vi "Main - Copy.vi"() -> ()   [LabVIEW 2017]
uses:
  <vilib>/addons/database/Connection.llb/Conn ObjectReference.ctl
  <vilib>/addons/database/Connection.llb/DB Tools Open Connec (Path).vi
  Globle/Current date.vi
  <vilib>/addons/database/Connection.llb/Conn Execute.vi
  <vilib>/addons/database/Recordset.llb/Rec Fetch Recordset Data (R).vi
  <vilib>/addons/database/Recordset.llb/Rec Destroy - Connection.vi
  <vilib>/addons/database/NI_Database_API.lvlib
  Globle/Stop.vi
panel:
  out "1D Array":string[](array[string])=["01:00 - 01:59", "02:00 - 02:59", "03:00 - 03:59", "04:00 - 04:59", "05:00 - 05:59", "06:00 - 06:59", "07:00 - 07:59", "08:00 - 08:59", "09:00 - 09:59", "10:00 - 10:59", "11:00 - 11:59", "12:00 - 12:59", "13:00 - 13:59", "14:00 - 14:59", "15:00 - 15:59", "16:00 - 16:59", "17:00 - 17:59", "18:00 - 18:59", "19:00 - 19:59", "20:00 - 20:59", "21:00 - 21:59", "22:00 - 22:59", "22:00 - 22:59", "00:00 - 01:59"]
  out "String Indicator 9":string="BREAKDOWN COUNT"
  out "String Indicator":string="PRODUCTION COUNT"
  out "String Indicator 8":string="REJECTION COUNT"
  out "Dlt Cnt":i32
  out "Table 2":string[][][](array[string])
  out "connection reference":T1
  out "String Indicator 7":string="RUNNING..."
  out "BDWn1":dbl
  out "Rej1":dbl
  out "Prod1":dbl
  out "Total Bdwn Time":timestamp format="%<%H:%M:%S>T"
  out "Hourly1":dbl[](array[numeric])
  out "BSWN3":dbl
  out "Rej3":dbl
  out "Prod 3":dbl
  out "Total Bdwn Time3":timestamp format="%<%H:%M:%S>T"
  out "String Indicator 3":string="RUNNING..."
  out "Hourly3":dbl[](array[numeric])
  out "BDWN2":dbl
  out "Rej2":dbl
  out "Prod 2":dbl
  out "Total Bdwn Time2":timestamp format="%<%H:%M:%S>T"
  out "String Indicator 2":string="RUNNING..."
  out "Hourly2":dbl[](array[numeric])
  out "BDWN6":dbl
  out "Rej6":dbl
  out "Prod6":dbl
  out "Total Bdwn Time4":timestamp format="%<%H:%M:%S>T"
  out "String Indicator 4":string="RUNNING..."
  out "Hourly6":dbl[](array[numeric])
  out "BDWN5":dbl
  out "Rej5":dbl
  out "Prod5":dbl
  out "Total Bdwn Time5":timestamp format="%<%H:%M:%S>T"
  out "String Indicator 5":string="RUNNING..."
  out "Hourly5":dbl[](array[numeric])
  out "BDWN4":dbl
  out "Rej4":dbl
  out "Prod4":dbl
  out "Total Bdwn Time6":timestamp format="%<%H:%M:%S>T"
  out "String Indicator 6":string="RUNNING..."
  out "Hourly4":dbl[](array[numeric])
  out "Numeric Indicator 4":string=" BREAKDOWN TIME "
  out "Numeric Indicator 3":string="STATUS"
  in  "Cancel Button - Archive":bool
  # "Main Screen"
  # "Station_1"
  # "Station_2"
  # "Station_3"
  # "Station_4"
  # "Station_5"
  # "Station_6"
  # "Designed & Developed By: Infinity Automation Systems Pvt. Ltd."
  # "00.00.53\n00.00.25\n00.00.21\n00.00.15\n11\n7\n2\n8\n1.6\n49\n35\n32\n27"
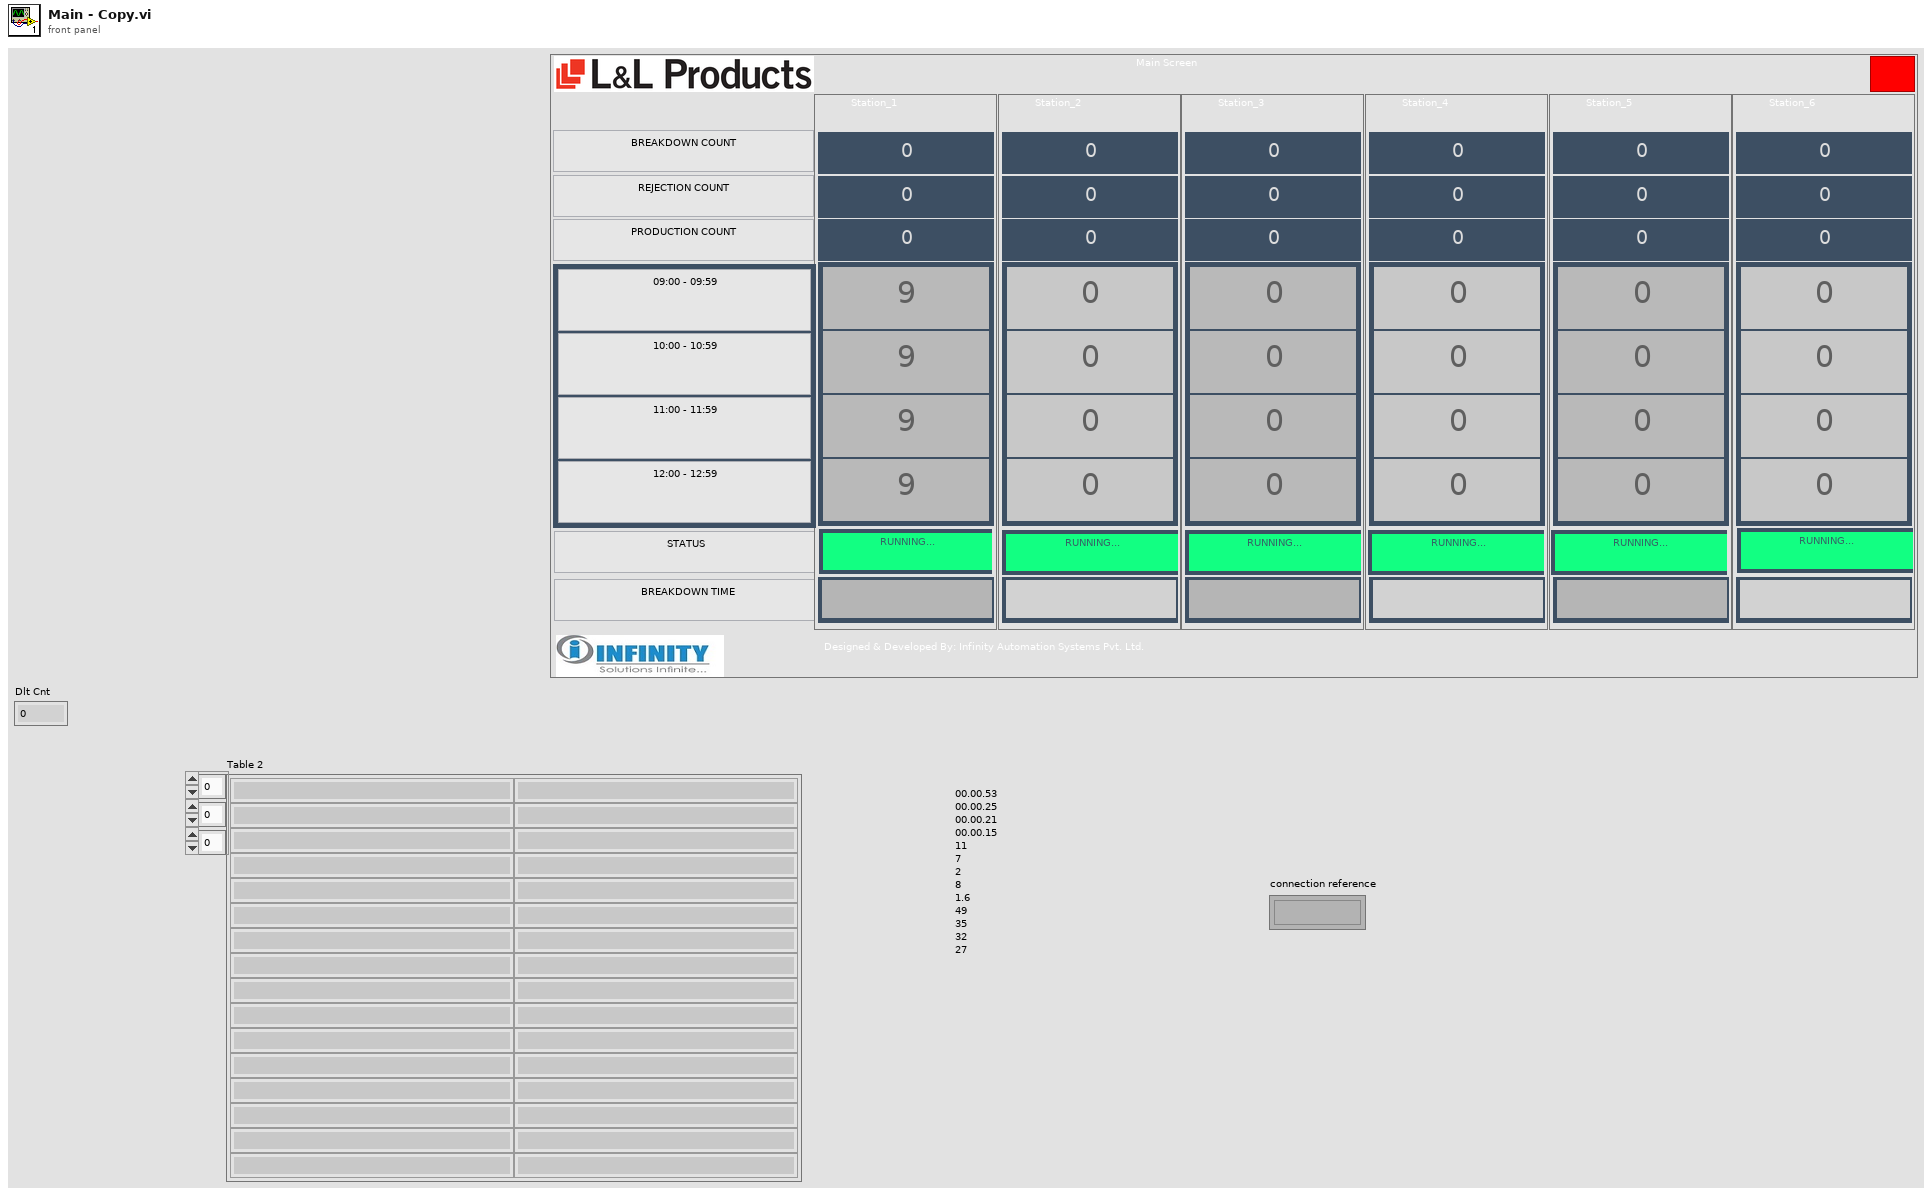
[diagram p1: front panel]
types:
  T1 = typedef "NI_Database_API.lvlib/Conn ObjectReference.ctl" = refnum<k1>
  T2 = typedef "NI_Database_API.lvlib/Rec ObjectReference.ctl" = refnum<k1>
  T3 = enum32{"invalid app kind", "Development System", "Run Time System", "Student Edition", "Embedded LabVIEW", "Evaluation", "Custom"}
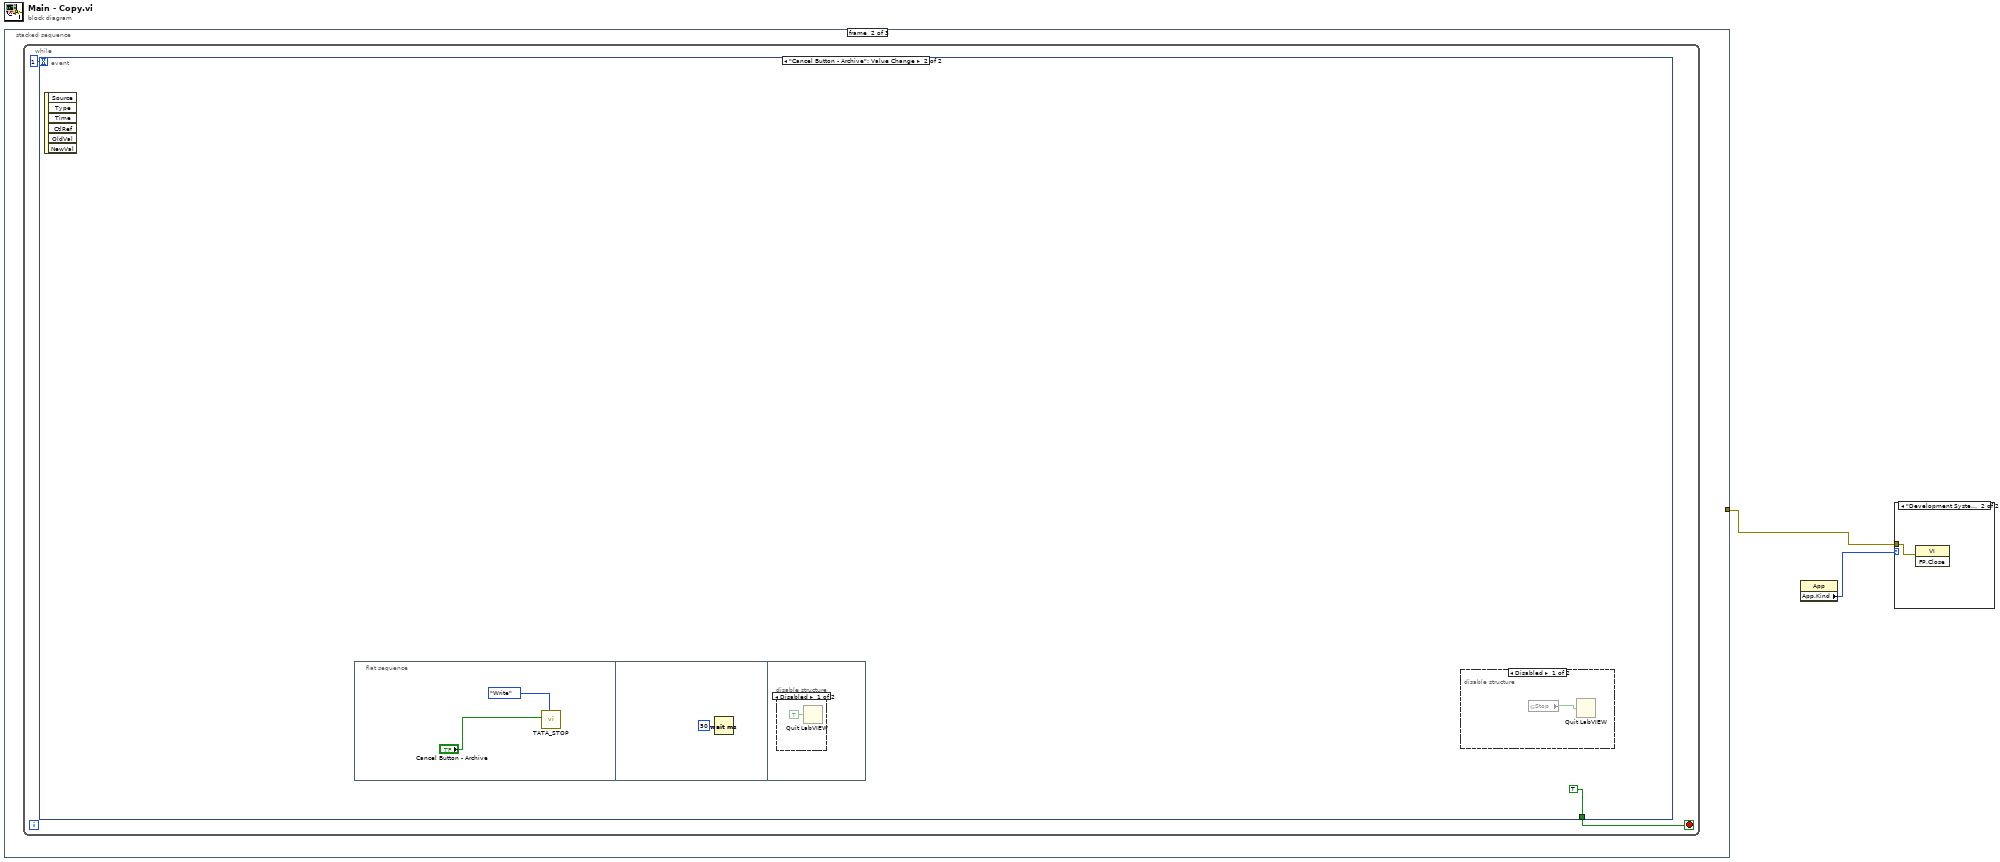
[diagram p0: block diagram]
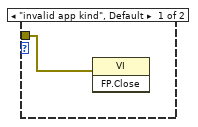
[diagram p2: hidden frame]
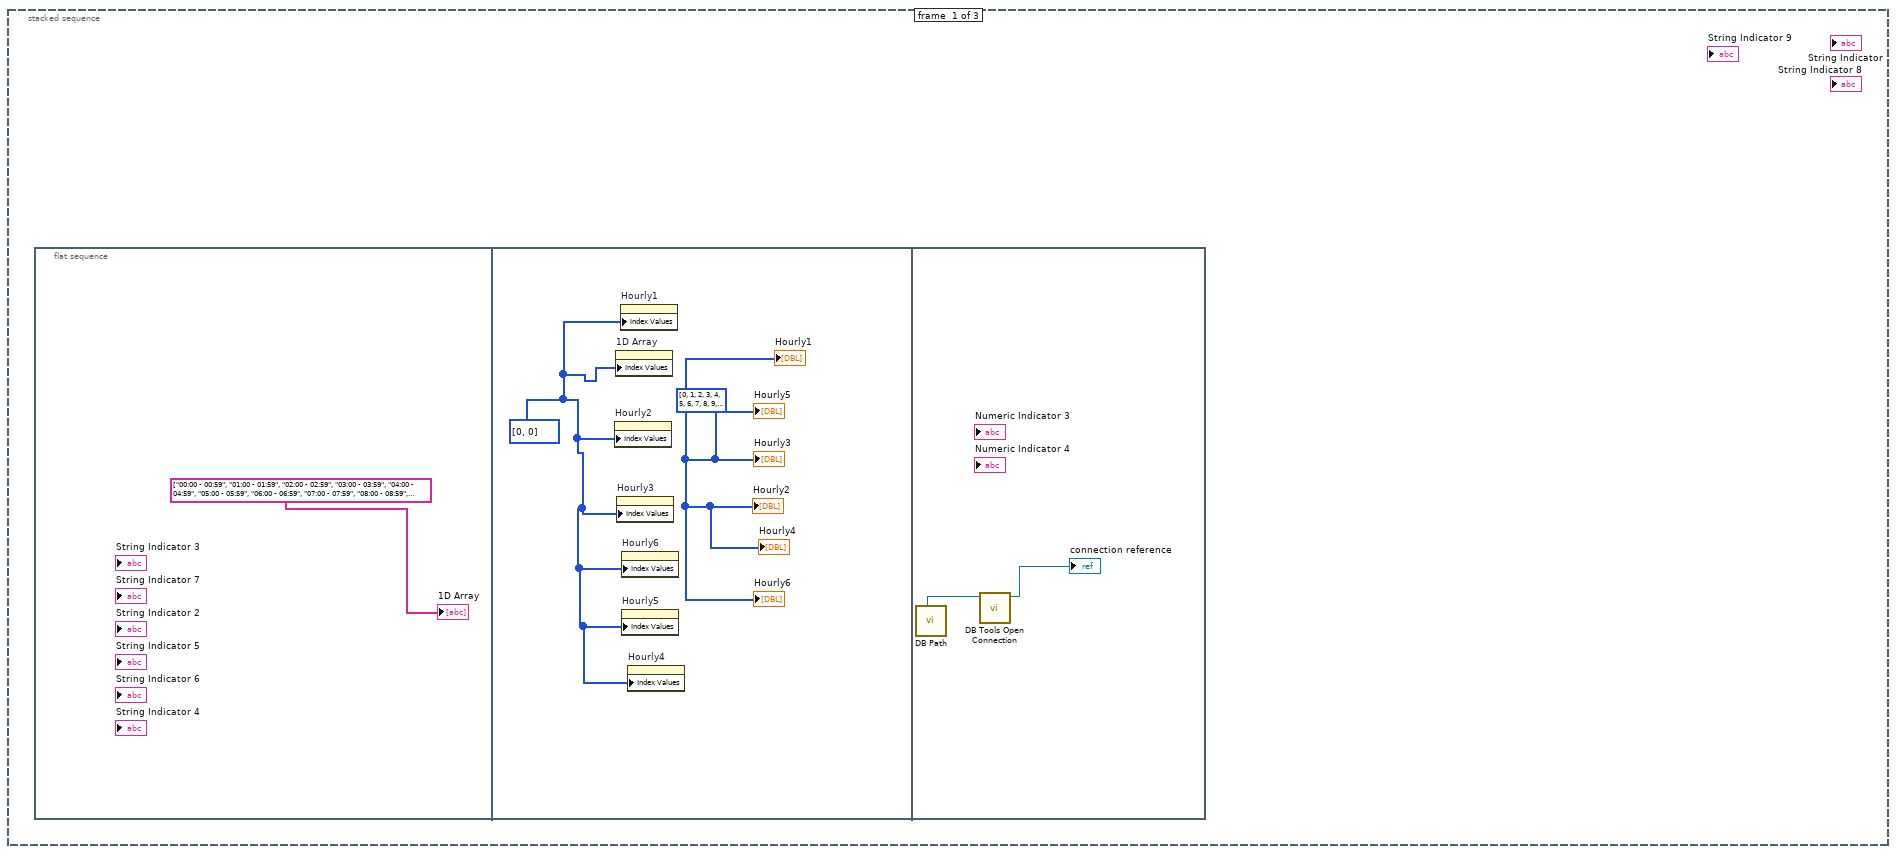
[diagram p3: hidden frame]
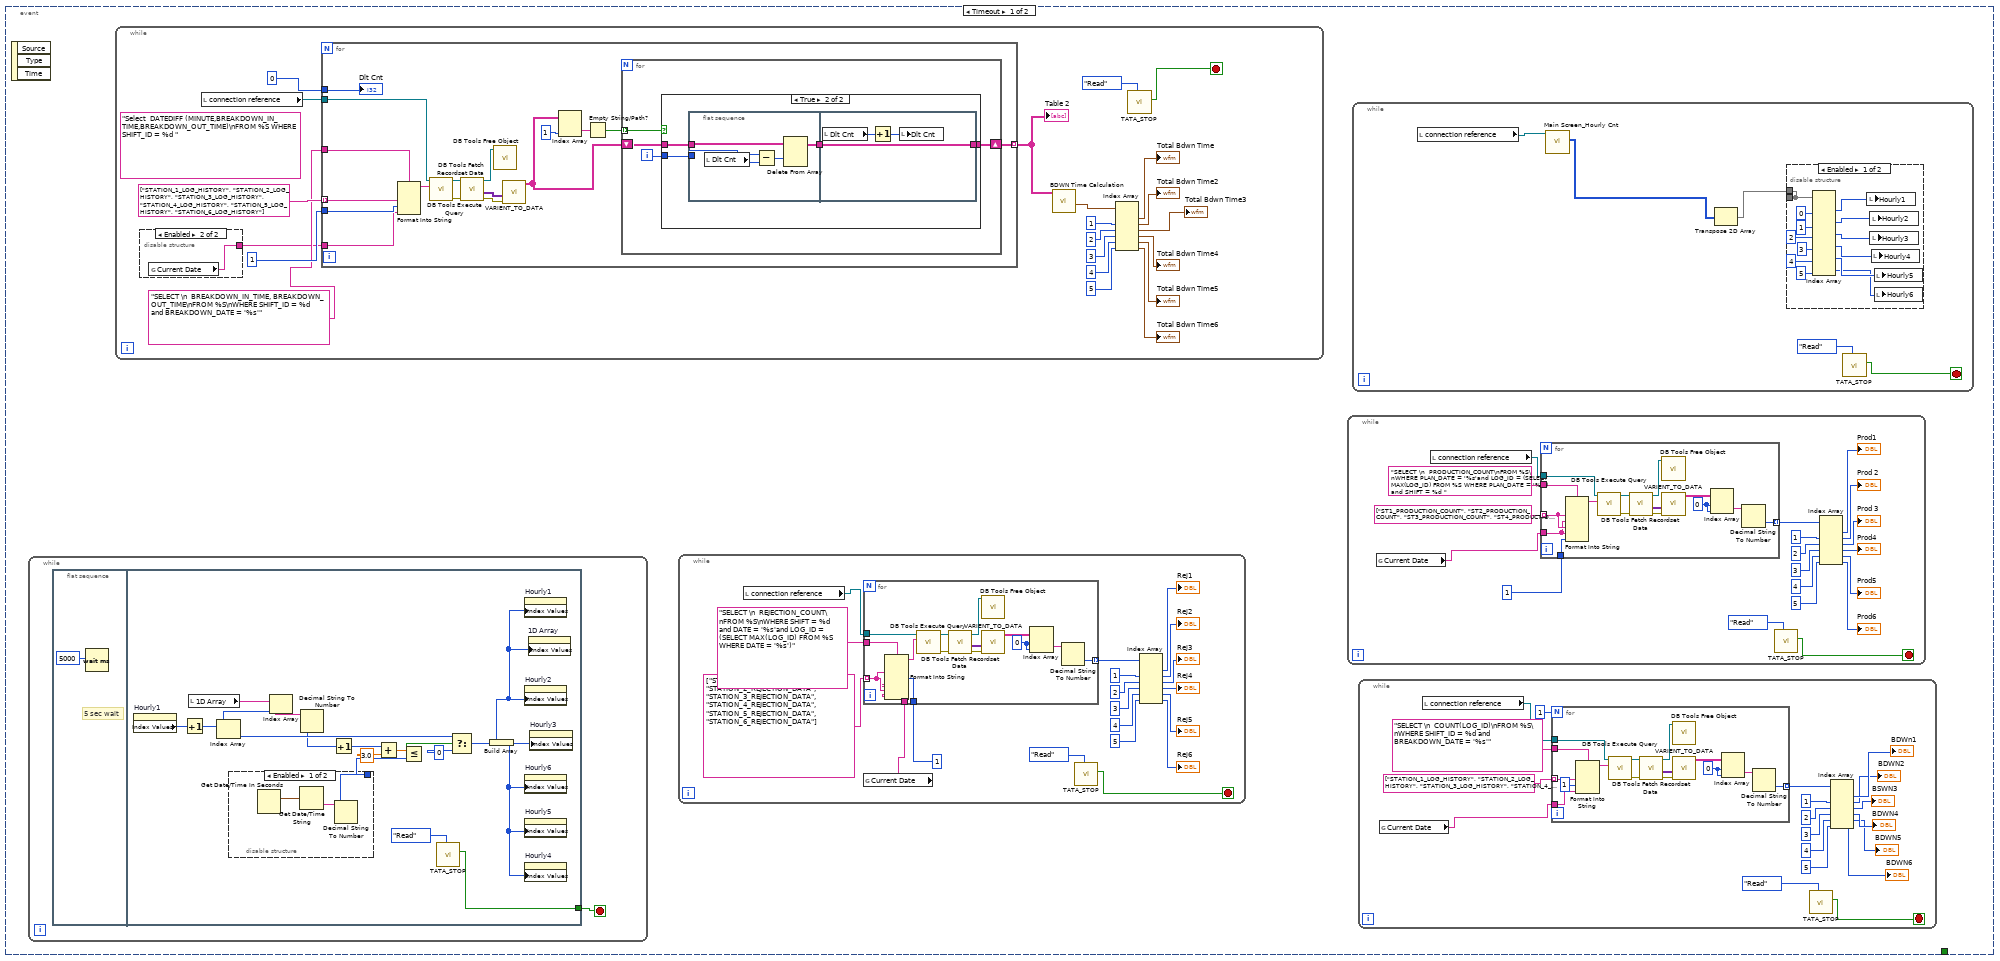
[diagram p4: hidden frame]
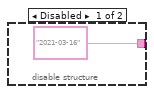
[diagram p6: hidden frame]
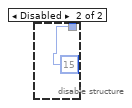
[diagram p8: hidden frame]
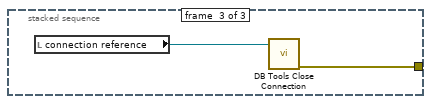
[diagram p11: hidden frame]
diagram:
  n1 = stacked-sequence {
    tunnel: [_ _ w215] -> w2
    frame #0 {
      n2 = flat-sequence {
        frame #0 {
          "1D Array" <- string[] ["00:00 - 00:59", "01:00 - 01:59", "02:00 - 02:59", "03:00 - 03:59", "04:00 - 04:59", "05:00 - 05:59", "06:00 - 06:59", "07:00 - 07:59", "08:00 - 08:59", "09:00 - 09:59", "10:00 - 10:59", "11:00 - 11:59", "12:00 - 12:59", "13:00 - 13:59", "14:00 - 14:59", "15:00 - 15:59", "16:00 - 16:59", "17:00 - 17:59", "18:00 - 18:59", "19:00 - 19:59", "20:00 - 20:59", "21:00 - 21:59", "22:00 - 22:59", "23:00 - 23:59"] ("array w/ subset deleted")
        }
        frame #1 {
          w5 = u32[] [0, 1, 2, 3, 4, 5, 6, 7, 8, 9, 10] ("appended array")
          w4 = u32[] [0, 0] ("appended array")
          n3 = property on="Hourly2" class="Arr (strict)"("Index Values"=w4) -> ()  [unwired: 2 in, 2 out]
          n4 = property on="1D Array" class="Arr (strict)"("Index Values"=w4) -> ()  [unwired: 2 in, 2 out]
          n5 = property on="Hourly3" class="Arr (strict)"("Index Values"=w4) -> ()  [unwired: 2 in, 2 out]
          n6 = property on="Hourly1" class="Arr (strict)"("Index Values"=w4) -> ()  [unwired: 2 in, 2 out]
          n7 = property on="Hourly6" class="Arr (strict)"("Index Values"=w4) -> ()  [unwired: 2 in, 2 out]
          n8 = property on="Hourly5" class="Arr (strict)"("Index Values"=w4) -> ()  [unwired: 2 in, 2 out]
          n9 = property on="Hourly4" class="Arr (strict)"("Index Values"=w4) -> ()  [unwired: 2 in, 2 out]
          "Hourly1" <- w5
          "Hourly5" <- w5
          "Hourly3" <- w5
          "Hourly2" <- w5
          "Hourly4" <- w5
          "Hourly6" <- w5
        }
        frame #2 {
          n10 = call "DB Path.vi"() -> ("DB Path"=w7:path)  [unwired: 10 in, 1 out]
          n11 = call-poly <vilib>:"DB Tools Open Connection.vi"("connection information"=w7) -> ("connection reference"=→"connection reference":T1)  [unwired: 7 in, 1 out]
        }
      }
    }
    frame #1 {
      n12 = while {
        stop <- w9 stop-if-true
        n13 = event shown="[1] \"Cancel Button - Archive\": Value Change" {
          selector: _ -> [_ _]
          dyn-events: _ -> [_ _]
          timeout: 1 -> [_ _]
          tunnel: [_ TRUE] -> w9
          event Timeout {
            n14 = event-data() -> ()  [unwired: 1 in, 3 out]
            n15 = while {
              stop <- w187 stop-if-true
              n16 = flat-sequence {
                tunnel: [w189] -> w187
                frame #0 {
                  # "5 sec wait"
                  n17 = Wait (ms)(milliseconds to wait=u32 5000) -> ()  [unwired: 1 out]
                }
                frame #1 {
                  n18 = property on="Hourly1" class="Arr (strict)"() -> ("Index Values"=w204:u32[])  [unwired: 2 in, 2 out]
                  n19 = Increment(x=w204) -> (x+1=w203:u32[])
                  n20 = local read "1D Array"() -> (w200:string[])
                  n21 = Index Array(array=w203) -> (element=w199:u32)  [unwired: 1 in]
                  n22 = disable-structure shown="Enabled" {
                    disable-tunnel: [w205 15] -> w195
                    frame Enabled {
                      n23 = Get Date/Time In Seconds() -> (seconds since 1Jan1904=w207:timestamp)
                      n24 = Get Date/Time String(seconds (now)=w207) -> (time string=w206:string)  [unwired: 2 in, 1 out]
                      n25 = Decimal String To Number(string=w206) -> (number=w205:i32)  [unwired: 2 in, 1 out]
                    }
                    frame Disabled {
                    }
                  }
                  n26 = Index Array(array=w200, index=w199) -> (element=w198:string)
                  n27 = Decimal String To Number(string=w198) -> (number=w197:i32)  [unwired: 2 in, 1 out]
                  n28 = Increment(x=w197) -> (x+1=w193:i32)
                  n29 = Add(x=w193, y=3.0) -> (x+y=w192:dbl)
                  n30 = Less Or Equal?(x=w192, y=w195) -> (x <= y?=w196:bool)
                  n31 = call "TATA_STOP.vi"("Enum"=enum16{"Read", "Write"}."Read") -> ("Boolean 2"=w189:bool)  [unwired: 9 in, 1 out]
                  n32 = Select(t=w199, s=w196, f=u32 0) -> (s? t:f=w201:u32)
                  n33 = Build Array(w201) -> (w191:u32[])
                  n34 = property on="Hourly1" class="Arr (strict)"("Index Values"=w191) -> ()  [unwired: 2 in, 2 out]
                  n35 = property on="Hourly2" class="Arr (strict)"("Index Values"=w191) -> ()  [unwired: 2 in, 2 out]
                  n36 = property on="Hourly6" class="Arr (strict)"("Index Values"=w191) -> ()  [unwired: 2 in, 2 out]
                  n37 = property on="Hourly5" class="Arr (strict)"("Index Values"=w191) -> ()  [unwired: 2 in, 2 out]
                  n38 = property on="Hourly4" class="Arr (strict)"("Index Values"=w191) -> ()  [unwired: 2 in, 2 out]
                  n39 = property on="1D Array" class="Arr (strict)"("Index Values"=w191) -> ()  [unwired: 2 in, 2 out]
                  n40 = property on="Hourly3" class="Arr (strict)"("Index Values"=w191) -> ()  [unwired: 2 in, 2 out]
                }
              }
            }
            n41 = while {
              stop <- w62 stop-if-true
              (unwired) "Select  DATEDIFF (MINUTE,BREAKDOWN_IN_TIME,BREAKDOWN_OUT_TIME)\nFROM %S WHERE SHIFT_ID = %d " ("SQL query")
              n42 = disable-structure shown="Enabled" {
                disable-tunnel: ["2021-03-16" w84] -> w64
                frame Disabled {
                }
                frame Enabled {
                  n43 = global read "Current date.vi" "Current Date"() -> (w84:string)
                }
              }
              n44 = local read "connection reference"() -> (w81:T1)
              n45 = for {
                tunnel: w81 -> [w101]
                tunnel: "SELECT \n  BREAKDOWN_IN_TIME, BREAKDOWN_OUT_TIME\nFROM %S\nWHERE SHIFT_ID = %d and BREAKDOWN_DATE = '%s'" ("SQL query") -> [w97]
                tunnel: string[] ["STATION_1_LOG_HISTORY", "STATION_2_LOG_HISTORY", "STATION_3_LOG_HISTORY", "STATION_4_LOG_HISTORY", "STATION_5_LOG_HISTORY", "STATION_6_LOG_HISTORY"] -> [w95] mode=indexing
                tunnel: 1 ("input 2") -> [w94]
                tunnel: 0 ("input 2") -> [w87]
                tunnel: [w86] -> w78 mode=indexing
                tunnel: w64 -> [w85]
                n46 = Format Into String(format string=w97, w95, w94, w85) -> (resulting string=w96:string)  [unwired: 2 in, 1 out]
                n47 = call-poly <vilib>:"DB Tools Execute Query.vi"("SQL query"=w96, "connection reference"=w101) -> ("error out"=w93:errorcluster, "recordset reference"=w100:T2)  [unwired: 6 in]
                n48 = call-poly <vilib>:"DB Tools Fetch Recordset Data.vi"("error in (no error)"=w93, "recordset reference"=w100) -> ("error out"=w92:errorcluster, "recordset data"=w98:variant[][], "recordset reference out"=w99:T2)  [unwired: 3 in]
                n49 = call-poly <vilib>:"DB Tools Free Object.vi"("recordset reference"=w99) -> ()  [unwired: 9 in, 2 out]
                n50 = call "VARIENT_TO_DATA.vi"("data"=w98, "error in (no error)"=w92) -> ("Table"=w88:string[][])  [unwired: 7 in, 1 out]
                n51 = Index Array(array=w88, index (col)=1 ("disabled index (col)")) -> (element=w90:string[])  [unwired: 1 in]
                n52 = Empty String/Path?(string/path=w90) -> (empty?=w89:bool[])
                n53 = for {
                  tunnel: w89 -> [w105] mode=indexing
                  shift-right: [w102] -> w86
                  shift-left: w88 -> [w104]
                  i -> [w103]
                  n54 = case shown="True" w105 {
                    tunnel: w104 -> [w106 w110]
                    tunnel: w103 -> [_ w109]
                    tunnel: [w106 w108] -> w102
                    frame False {
                    }
                    frame True {
                      n55 = flat-sequence {
                        tunnel: w110 -> [w115]
                        tunnel: w109 -> [w113]
                        tunnel: [w114] -> w107
                        tunnel: [w118] -> w108
                        tunnel: w107 -> [w118]
                        frame #0 {
                          n56 = local read "Dlt Cnt"() -> (w112:i32)
                          n57 = Subtract(x=w113, y=w112) -> (x-y=w111:i32)
                          n58 = Delete From Array(array=w115, index (row)=w111) -> (array with subset deleted=w114:string[][])  [unwired: 2 in, 1 out]
                        }
                        frame #1 {
                          n59 = local read "Dlt Cnt"() -> (w116:i32)
                          n60 = Increment(x=w116) -> (x+1=w117:i32)
                          n61 = local write "Dlt Cnt"(w117) -> ()
                        }
                      }
                    }
                  }
                }
                "Dlt Cnt" <- w87
              }
              "Table 2" <- w78
              n62 = call "BDWN Time Calculation.vi"("Input Table"=w78) -> ("All BDWN Time"=w77:timestamp[])  [unwired: 8 in, 1 out]
              n63 = Index Array(array=w77, index #2=1 ("index"), index #3=2 ("index"), index #4=3 ("index"), index #5=4 ("index"), index #6=5 ("index")) -> (element #1=→"Total Bdwn Time":timestamp, element #2=→"Total Bdwn Time2":timestamp, element #3=→"Total Bdwn Time3":timestamp, element #4=→"Total Bdwn Time4":timestamp, element #5=→"Total Bdwn Time5":timestamp, element #6=→"Total Bdwn Time6":timestamp)  [unwired: 1 in]
              n64 = call "TATA_STOP.vi"("Enum"=enum16{"Read", "Write"}."Read") -> ("Boolean 2"=w62:bool)  [unwired: 9 in, 1 out]
            }
            n65 = while {
              stop <- w153 stop-if-true
              n66 = local read "connection reference"() -> (w157:T1)
              n67 = global read "Current date.vi" "Current Date"() -> (w155:string)
              n68 = for {
                tunnel: w157 -> [w186]
                tunnel: "SELECT \n  REJECTION_COUNT\nFROM %S\nWHERE SHIFT = %d and DATE = '%s'and LOG_ID = (SELECT MAX(LOG_ID) FROM %S WHERE DATE = '%s')" ("SQL query") -> [w182]
                tunnel: string[] ["STATION_1_REJECTION_DATA", "STATION_2_REJECTION_DATA", "STATION_3_REJECTION_DATA", "STATION_4_REJECTION_DATA", "STATION_5_REJECTION_DATA", "STATION_6_REJECTION_DATA"] -> [w174] mode=indexing
                tunnel: [w177] -> w169 mode=indexing
                tunnel: w155 -> [w172]
                tunnel: 1 ("index") -> [w173]
                w179 = 0 ("index (row)")
                n69 = Format Into String(format string=w182, w174, w173, w172, w174, w172) -> (resulting string=w181:string)  [unwired: 2 in, 1 out]
                n70 = call-poly <vilib>:"DB Tools Execute Query.vi"("SQL query"=w181, "connection reference"=w186) -> ("error out"=w176:errorcluster, "recordset reference"=w185:T2)  [unwired: 6 in]
                n71 = call-poly <vilib>:"DB Tools Fetch Recordset Data.vi"("error in (no error)"=w176, "recordset reference"=w185) -> ("error out"=w175:errorcluster, "recordset data"=w183:variant[][], "recordset reference out"=w184:T2)  [unwired: 3 in]
                n72 = call-poly <vilib>:"DB Tools Free Object.vi"("recordset reference"=w184) -> ()  [unwired: 9 in, 2 out]
                n73 = call "VARIENT_TO_DATA.vi"("data"=w183, "error in (no error)"=w175) -> ("Table"=w180:string[][])  [unwired: 7 in, 1 out]
                n74 = Index Array(array=w180, index (row)=w179, index (col)=w179) -> (element=w178:string)
                n75 = Decimal String To Number(string=w178) -> (number=w177:i32)  [unwired: 2 in, 1 out]
              }
              n76 = call "TATA_STOP.vi"("Enum"=enum16{"Read", "Write"}."Read") -> ("Boolean 2"=w153:bool)  [unwired: 9 in, 1 out]
              n77 = Index Array(array=w169, index #2=1 ("index"), index #3=2 ("index"), index #4=3 ("index"), index #5=4 ("index"), index #6=5 ("index")) -> (element #1=→"Rej1":i32, element #2=→"Rej2":i32, element #3=→"Rej3":i32, element #4=→"Rej4":i32, element #5=→"Rej5":i32, element #6=→"Rej6":i32)  [unwired: 1 in]
            }
            n78 = while {
              stop <- w119 stop-if-true
              n79 = global read "Current date.vi" "Current Date"() -> (w121:string)
              n80 = local read "connection reference"() -> (w123:T1)
              n81 = for {
                tunnel: w123 -> [w152]
                tunnel: "SELECT \n  PRODUCTION_COUNT\nFROM %S\nWHERE PLAN_DATE = '%s'and LOG_ID = (SELECT MAX(LOG_ID) FROM %S WHERE PLAN_DATE = '%s') and SHIFT = %d " ("SQL query") -> [w148]
                tunnel: string[] ["ST1_PRODUCTION_COUNT", "ST2_PRODUCTION_COUNT", "ST3_PRODUCTION_COUNT", "ST4_PRODUCTION_COUNT", "ST5_PRODUCTION_COUNT", "ST6_PRODUCTION_COUNT"] -> [w140] mode=indexing
                tunnel: [w143] -> w135 mode=indexing
                tunnel: w121 -> [w139]
                tunnel: 1 ("index") -> [w138]
                w145 = 0 ("index (row)")
                n82 = Format Into String(format string=w148, w140, w139, w140, w139, w138) -> (resulting string=w147:string)  [unwired: 2 in, 1 out]
                n83 = call-poly <vilib>:"DB Tools Execute Query.vi"("SQL query"=w147, "connection reference"=w152) -> ("error out"=w142:errorcluster, "recordset reference"=w151:T2)  [unwired: 6 in]
                n84 = call-poly <vilib>:"DB Tools Fetch Recordset Data.vi"("error in (no error)"=w142, "recordset reference"=w151) -> ("error out"=w141:errorcluster, "recordset data"=w149:variant[][], "recordset reference out"=w150:T2)  [unwired: 3 in]
                n85 = call-poly <vilib>:"DB Tools Free Object.vi"("recordset reference"=w150) -> ()  [unwired: 9 in, 2 out]
                n86 = call "VARIENT_TO_DATA.vi"("data"=w149, "error in (no error)"=w141) -> ("Table"=w146:string[][])  [unwired: 7 in, 1 out]
                n87 = Index Array(array=w146, index (row)=w145, index (col)=w145) -> (element=w144:string)
                n88 = Decimal String To Number(string=w144) -> (number=w143:i32)  [unwired: 2 in, 1 out]
              }
              n89 = call "TATA_STOP.vi"("Enum"=enum16{"Read", "Write"}."Read") -> ("Boolean 2"=w119:bool)  [unwired: 9 in, 1 out]
              n90 = Index Array(array=w135, index #2=1 ("index"), index #3=2 ("index"), index #4=3 ("index"), index #5=4 ("index"), index #6=5 ("index")) -> (element #1=→"Prod1":i32, element #2=→"Prod 2":i32, element #3=→"Prod 3":i32, element #4=→"Prod4":i32, element #5=→"Prod5":i32, element #6=→"Prod6":i32)  [unwired: 1 in]
            }
            n91 = while {
              stop <- w44 stop-if-true
              n92 = local read "connection reference"() -> (w48:T1)
              n93 = call "Main Screen_Hourly Cnt.vi"("connection reference 2"=w48) -> ("Station Wise Max"=w47:i32[][])  [unwired: 10 in]
              n94 = Transpose 2D Array(2D array=w47) -> (transposed array=w46:i32[][])
              n95 = disable-structure shown="Enabled" {
                disable-tunnel: [w49 _] -> _
                disable-tunnel: w46 -> [w49 _]
                frame Enabled {
                  n96 = Index Array(array=w49, index (col) #1=0 ("disabled index (col)"), index (col) #2=1 ("index (col)"), index (col) #3=2 ("index (col)"), index (col) #4=3 ("index (col)"), index (col) #5=4 ("index (col)"), index (col) #6=5 ("index (col)")) -> (element #1=w55:i32[], element #2=w54:i32[], element #3=w53:i32[], element #4=w52:i32[], element #5=w51:i32[], element #6=w50:i32[])  [unwired: 6 in]
                  n97 = local write "Hourly1"(w55) -> ()
                  n98 = local write "Hourly2"(w54) -> ()
                  n99 = local write "Hourly3"(w53) -> ()
                  n100 = local write "Hourly4"(w52) -> ()
                  n101 = local write "Hourly5"(w51) -> ()
                  n102 = local write "Hourly6"(w50) -> ()
                }
                frame Disabled {
                }
              }
              n103 = call "TATA_STOP.vi"("Enum"=enum16{"Read", "Write"}."Read") -> ("Boolean 2"=w44:bool)  [unwired: 9 in, 1 out]
            }
            n104 = while {
              stop <- w11 stop-if-true
              n105 = global read "Current date.vi" "Current Date"() -> (w14:string)
              n106 = local read "connection reference"() -> (w22:T1)
              n107 = for {
                N: 1 -> [_]
                tunnel: w22 -> [w43]
                tunnel: "SELECT \n  COUNT(LOG_ID)\nFROM %S\nWHERE SHIFT_ID = %d and BREAKDOWN_DATE = '%s'" ("SQL query") -> [w39]
                tunnel: string[] ["STATION_1_LOG_HISTORY", "STATION_2_LOG_HISTORY", "STATION_3_LOG_HISTORY", "STATION_4_LOG_HISTORY", "STATION_5_LOG_HISTORY", "STATION_6_LOG_HISTORY"] -> [w31] mode=indexing
                tunnel: [w34] -> w27 mode=indexing
                tunnel: w14 -> [w30]
                w36 = 0 ("index (row)")
                n108 = Format Into String(format string=w39, w31, 1 ("input 2"), w30) -> (resulting string=w38:string)  [unwired: 2 in, 1 out]
                n109 = call-poly <vilib>:"DB Tools Execute Query.vi"("SQL query"=w38, "connection reference"=w43) -> ("error out"=w33:errorcluster, "recordset reference"=w42:T2)  [unwired: 6 in]
                n110 = call-poly <vilib>:"DB Tools Fetch Recordset Data.vi"("error in (no error)"=w33, "recordset reference"=w42) -> ("error out"=w32:errorcluster, "recordset data"=w40:variant[][], "recordset reference out"=w41:T2)  [unwired: 3 in]
                n111 = call-poly <vilib>:"DB Tools Free Object.vi"("recordset reference"=w41) -> ()  [unwired: 9 in, 2 out]
                n112 = call "VARIENT_TO_DATA.vi"("data"=w40, "error in (no error)"=w32) -> ("Table"=w37:string[][])  [unwired: 7 in, 1 out]
                n113 = Index Array(array=w37, index (row)=w36, index (col)=w36) -> (element=w35:string)
                n114 = Decimal String To Number(string=w35) -> (number=w34:i32)  [unwired: 2 in, 1 out]
              }
              n115 = call "TATA_STOP.vi"("Enum"=enum16{"Read", "Write"}."Read") -> ("Boolean 2"=w11:bool)  [unwired: 9 in, 1 out]
              n116 = Index Array(array=w27, index #2=1 ("index"), index #3=2 ("index"), index #4=3 ("index"), index #5=4 ("index"), index #6=5 ("index")) -> (element #1=→"BDWn1":i32, element #2=→"BDWN2":i32, element #3=→"BSWN3":i32, element #4=→"BDWN4":i32, element #5=→"BDWN5":i32, element #6=→"BDWN6":i32)  [unwired: 1 in]
            }
          }
          event "Cancel Button - Archive": Value Change {
            n117 = event-data() -> ()  [unwired: 1 in, 6 out]
            n118 = flat-sequence {
              frame #0 {
                n119 = call "TATA_STOP.vi"("Enum"=enum16{"Read", "Write"}."Write", "Boolean"="Cancel Button - Archive") -> ()  [unwired: 8 in, 2 out]
              }
              frame #1 {
                n120 = Wait (ms)(milliseconds to wait=u32 50) -> ()  [unwired: 1 out]
              }
              frame #2 {
                n121 = disable-structure shown="Disabled" {
                  frame Disabled {
                    n122 = Quit LabVIEW(quit? (T)=TRUE) -> ()
                  }
                  frame Enabled {
                  }
                }
              }
            }
            n123 = disable-structure shown="Disabled" {
              frame Disabled {
                n124 = global read "Stop.vi" "Stop"() -> (w214:bool)
                n125 = Quit LabVIEW(quit? (T)=w214) -> ()
              }
              frame Enabled {
              }
            }
          }
        }
      }
    }
    frame #2 {
      n126 = local read "connection reference"() -> (w216:T1)
      n127 = call <vilib>:"DB Tools Close Connection.vi"("connection reference"=w216) -> ("error out"=w215:errorcluster)  [unwired: 6 in]
    }
  }
  n128 = property class="App"() -> ("App.Kind"=w1:T3)  [unwired: 2 in, 2 out]
  n129 = case shown="\"Development System\"" w1 {
    tunnel: w2 -> [w217 w218]
    frame "invalid app kind", Default {
      n130 = invoke class="VI" method="FP.Close"(error in=w217) -> ()  [unwired: 2 in, 3 out]
    }
    frame "Development System" {
      n131 = invoke class="VI" method="FP.Close"(error in=w218) -> ()  [unwired: 2 in, 3 out]
    }
  }
